vi "Write Packet.vi"(0 "comm interface in":refnum<class "Pixy Com.lvclass">, 5 "type":u8, 7 "payload":u8[](array[numeric]), 11 "error in":errorcluster) -> (4 "comm interface out":refnum<class "Pixy Com.lvclass">, 15 "error out":errorcluster)   [LabVIEW 2018, in "Pixy2.lvlib"]
uses:
  Pixy2.lvlib
  Interface/Pixy Com.lvclass
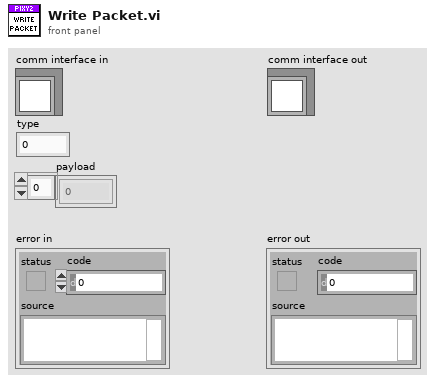
[diagram p1: front panel]
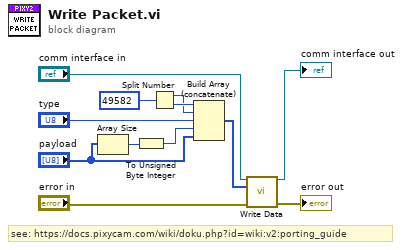
[diagram p0: block diagram]
diagram:
  # "see: https://docs.pixycam.com/wiki/doku.php?id=wiki:v2:porting_guide"
  n1 = Array Size(array="payload") -> (size(s)=w12:i32)
  n2 = To Unsigned Byte Integer(number=w12) -> (unsigned 8bit integer=w11:u8)
  n3 = Split Number(x=u16 49582) -> (hi(x)=w4:u8, lo(x)=w5:u8)
  n4 = Build Array (concatenate)(w5, w4, "type", w11, "payload") -> (w10:u8[])
  n5 = call-dynamic "Write Data.vi"("comm interface in"="comm interface in", "data"=w10, "error in"="error in") -> ("comm interface out"=→"comm interface out":refnum<class "Pixy Com.lvclass">, "error out"=→"error out":errorcluster)  [unwired: 11 in]
